vi "Simple Y16 Picture.vi"() -> ()   [LabVIEW 2020]
panel:
  in  "ICImagingControl":refnum<k7>(container)
  out "Error Out":errorcluster
  out "Picture Out":picture
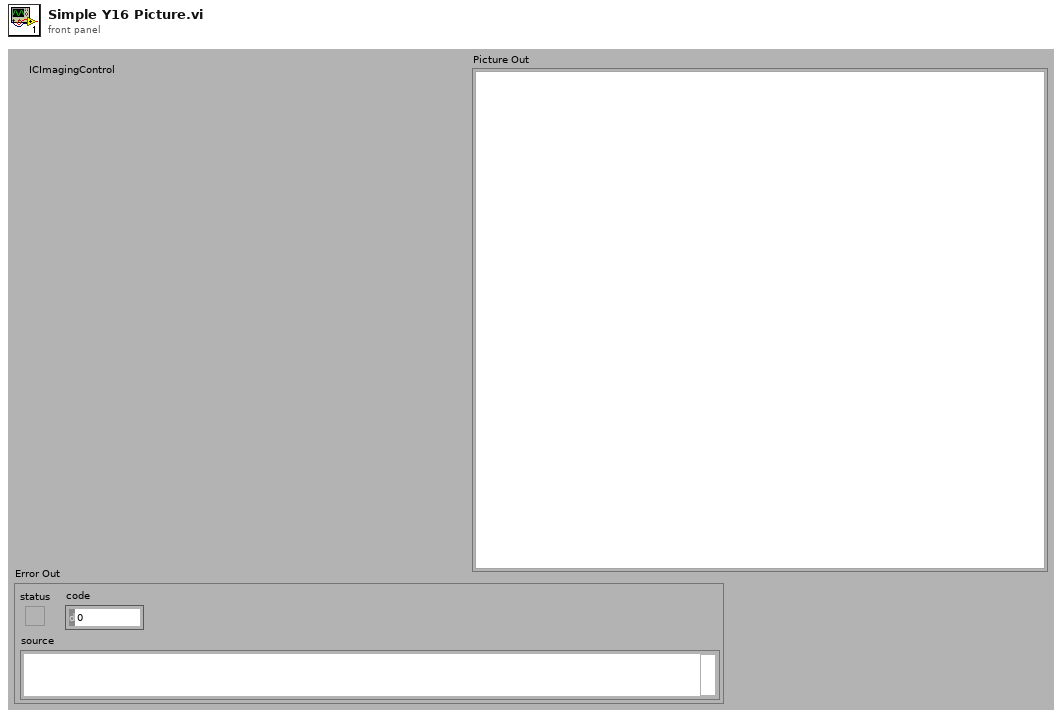
[diagram p1: front panel]
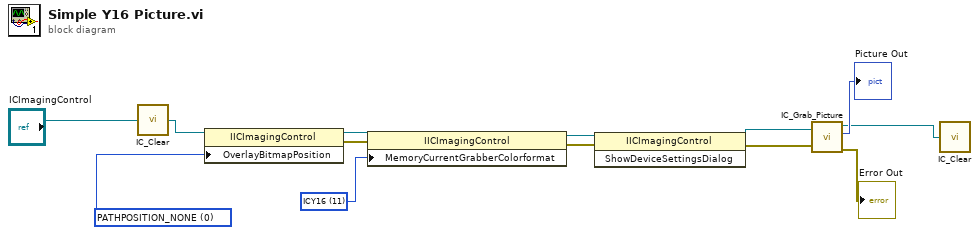
[diagram p0: block diagram]
diagram:
  w13 = 0 items=["PATHPOSITION_NONE"=0, "PATHPOSITION_DEVICE"=1, "PATHPOSITION_SINK"=2, "PATHPOSITION_DISPLAY"=4] ("OverlayBitmapPosition")
  w10 = 11 items=["ICRGB32"=1, "ICRGB24"=2, "ICRGB565"=3, "ICRGB555"=4, "ICY8"=5, "ICUYVY"=6, "ICY800"=7, "ICYGB1"=8, "ICYGB0"=9, "ICBY8"=10, "ICY16"=11] ("MemoryCurrentGrabberColorformat")
  n1 = call "IC_Clear.vi"("ICImagingControl 2"="ICImagingControl") -> ("ICImagingControl"=w9:refnum<k7>)
  n2 = property class="IICImagingControl"(reference=w9, "OverlayBitmapPosition"=w13) -> (reference out=w7:refnum<k7>, error out=w4:errorcluster)  [unwired: 1 in]
  n3 = property class="IICImagingControl"(reference=w7, error in=w4, "MemoryCurrentGrabberColorformat"=w10) -> (reference out=w6:refnum<k7>, error out=w3:errorcluster)
  n4 = invoke class="IICImagingControl" method="ShowDeviceSettingsDialog"(reference=w6, error in=w3) -> (reference out=w5:refnum<k7>, error out=w2:errorcluster)  [unwired: 1 in, 1 out]
  n5 = call "IC_Grab_Picture.vi"("ICImagingControl In"=w5, "Error In (no error)"=w2) -> ("ICImagingControl Out"=w8:refnum<k7>, "Picture Out"=→"Picture Out":picture, "Error Out"=→"Error Out":errorcluster)  [unwired: 1 out]
  n6 = call "IC_Clear.vi"("ICImagingControl 2"=w8) -> ()  [unwired: 1 out]
